vi "Quick Start - Simple - Create Data Source.vi"() -> ()   [LabVIEW 2020]
uses:
  Nominal Client/Nominal Client.lvclass/Nominal Client.ctl
  48e63680-6a8c-4ade-94df-21daa40b76be.vi
  Nominal Client/private_data.set.vi
  <vilib>/Utility/file.llb/Application Directory.vi
  <vilib>/Utility/error.llb/Error Cluster From Error Code.vi
  submodules/reqwest-labview/lv-src/reqwest/create.vi
  Nominal Client/Nominal Client.lvclass
  nominal types/workspace/workspace.lvclass
  submodules/reqwest-labview/lv-src/reqwest/reqwest.lvclass
panel:
  out "Created Data Source":T1
  out "rid":string
  in  "Description":string
  in  "ID":string
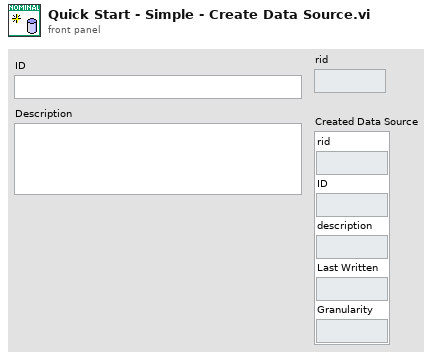
[diagram p1: front panel]
types:
  T1 = cluster{"rid":string, "ID":string, "description":string, "Last Written":string, "Granularity":string}
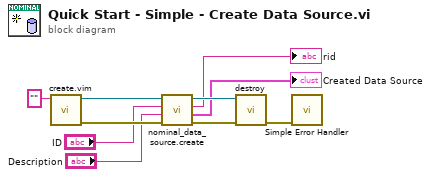
[diagram p0: block diagram]
diagram:
  n1 = call "create.vim"("API Token (string or path)"="") -> ("error out"=w9:errorcluster, "Nominal Client"=w10:refnum<class "Nominal Client.lvclass">)  [unwired: 9 in]
  n2 = call "nominal_data_source.create.vi"("error in"=w9, "Description"="Description", "Name"="ID", "Nominal Client in"=w10) -> ("error out"=w7:errorcluster, "Created Data Source"=→"Created Data Source":T1, "rid"=→"rid":string, "Nominal Client out"=w8:refnum<class "Nominal Client.lvclass">)  [unwired: 4 in]
  n3 = call "destroy.vi"("error in"=w7, "Nominal Client"=w8) -> ("error out"=w3:errorcluster)  [unwired: 9 in]
  n4 = call <vilib>:"Simple Error Handler.vi"("error in (no error)"=w3) -> ()  [unwired: 4 in, 5 out]
